vi "InterfaceAODSWWithStabilizationSW.vi"(8 "Grid Points":dbl, 9 "Motion Points":dbl, 10 "Channel":i32, 11 "Data":waveform(i32)[](array[waveform])) -> (2 "Number of Planes":dbl, 3 "Array":cluster{dbl[][], dbl, dbl, dbl, dbl, dbl, dbl}[](array[cluster]))   [LabVIEW 2011]
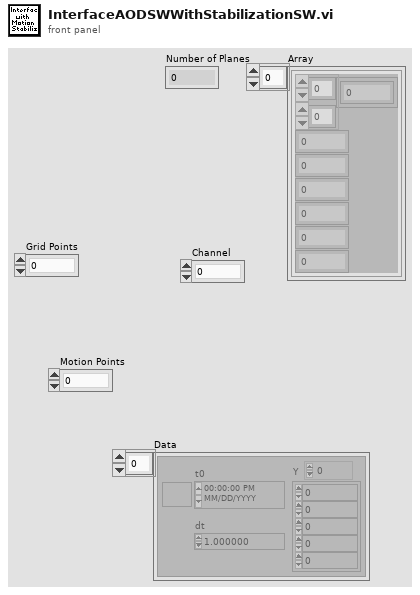
[diagram p1: front panel]
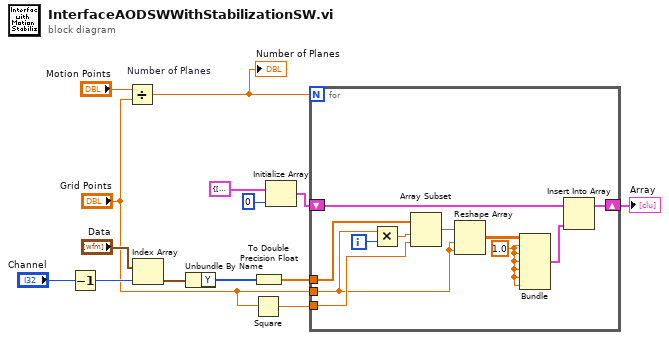
[diagram p0: block diagram]
diagram:
  n1 = Decrement(x="Channel") -> (x-1=w12:i32)
  n2 = Divide "Number of Planes"(x="Motion Points", y="Grid Points") -> (x/y=w10:dbl)
  "Number of Planes" <- w10
  n3 = Index Array(array="Data", index=w12) -> (element=w11:waveform(i32))
  n4 = Unbundle By Name(w11) -> ("Y"=w7:i32[])
  n5 = Square(x="Grid Points") -> (x^2=w9:dbl)
  n6 = To Double Precision Float(number=w7) -> (double precision float=w6:dbl[])
  n7 = Initialize Array(cluster{dbl[][], dbl, dbl, dbl, dbl, dbl, dbl} {[], 0.0, 0.0, 0.0, 0.0, 0.0, 0.0} ("output cluster"), 0 ("dimension size")) -> (w4:cluster{dbl[][], dbl, dbl, dbl, dbl, dbl, dbl}[])
  n8 = for {
    N: w10 -> [_]
    tunnel: w6 -> [w25]
    tunnel: "Grid Points" -> [w20]
    tunnel: w9 -> [w22]
    shift-right: [w15] -> w1
    shift-left: w4 -> [w16]
    i -> [w23]
    w19 = 1.0
    n9 = Multiply(x=w20, y=w23) -> (x*y=w24:dbl)
    n10 = Array Subset(array=w25, index=w24, length=w22) -> (w21:dbl[])
    n11 = Reshape Array(w21, w20, w20) -> (w18:dbl[][])
    n12 = Bundle(w18, w19, w19, w19, w19, w19, w19) -> (w17:cluster{dbl[][], dbl, dbl, dbl, dbl, dbl, dbl})  [unwired: 1 in]
    n13 = Insert Into Array(array=w16, new element=w17) -> (w15:cluster{dbl[][], dbl, dbl, dbl, dbl, dbl, dbl}[])  [unwired: 1 in]
  }
  "Array" <- w1
